vi "Extract Signal Bits.vi"(11 "Test Case In":refnum<class "test CAN Frame.lvclass">) -> (0 "error out":errorcluster, 3 "Test Case Out":refnum<class "test CAN Frame.lvclass">)   [LabVIEW 2023, in "test CAN Frame.lvclass"]
uses:
  test CAN Frame.lvclass
  test CAN Frame.lvclass/test CAN Frame.ctl
  4993e8ee-a06a-463a-9684-69129f64d5ce.vi
  CAN Frame/CAN Frame.lvclass
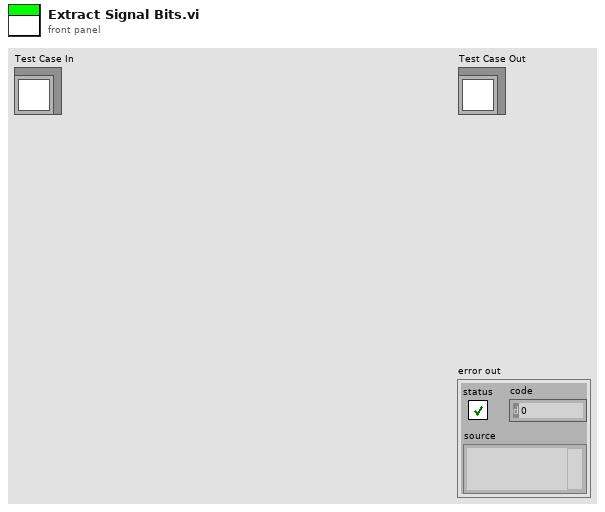
[diagram p1: front panel]
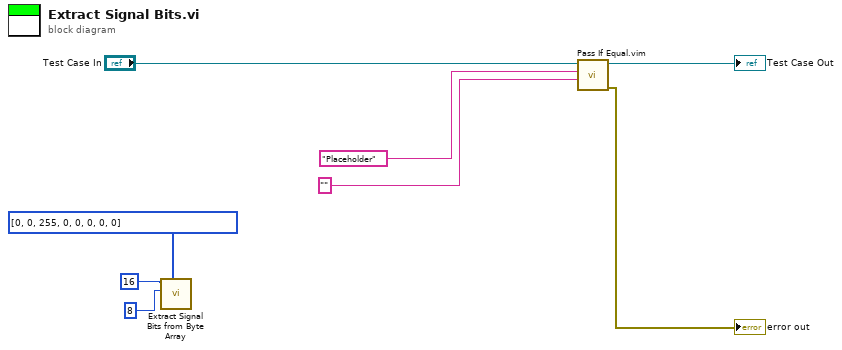
[diagram p0: block diagram]
diagram:
  n1 = call "Extract Signal Bits from Byte Array.vi"("Payload"=u8[] [0, 0, 255, 0, 0, 0, 0, 0], "Bit Length"=u32 8, "Start Bit"=u32 16) -> ()  [unwired: 8 in, 1 out]
  n2 = call "Pass If Equal.vim"("Actual"="", "Expected"="Placeholder", "LUnit Test Case In"="Test Case In") -> ("error out"=→"error out":errorcluster, "LUnit Test Case Out"=→"Test Case Out":refnum<class "test CAN Frame.lvclass">)  [unwired: 7 in]
